vi "读取反控数据解析(子VI).vi"(6 "数据":string, 7 "命令编码CN":string) -> (0 "实时数据发送时间间隔/min":i32=1, 2 "设置超时时间/min":i32=1, 3 "反控命令错误？":bool)   [LabVIEW 2016, in "数据传输系统.lvlib"]
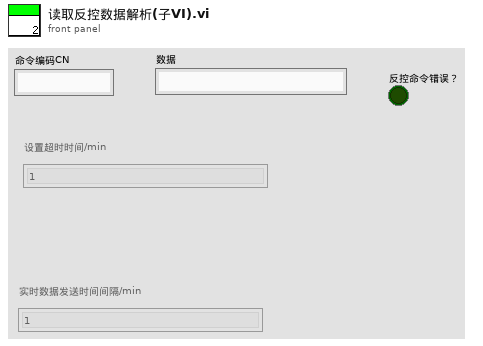
[diagram p1: front panel]
types:
  T1 = enum16{"初始化", "打开连接", "表格比对", "发送数据", "读取数据", "数据处理"}
  T2 = enum16{"CODMn", "CODCr", "氨氮", "总磷", "总氮", "数采仪"}
  T3 = cluster{"高锰酸盐":string, "化学需氧量":string, "氨氮":string, "总磷":string, "总氮":string, "数采仪":string, "高锰酸盐":bool, "化学需氧量":bool, "氨氮":bool, "总磷":bool, "总氮":bool, "数采仪":bool}
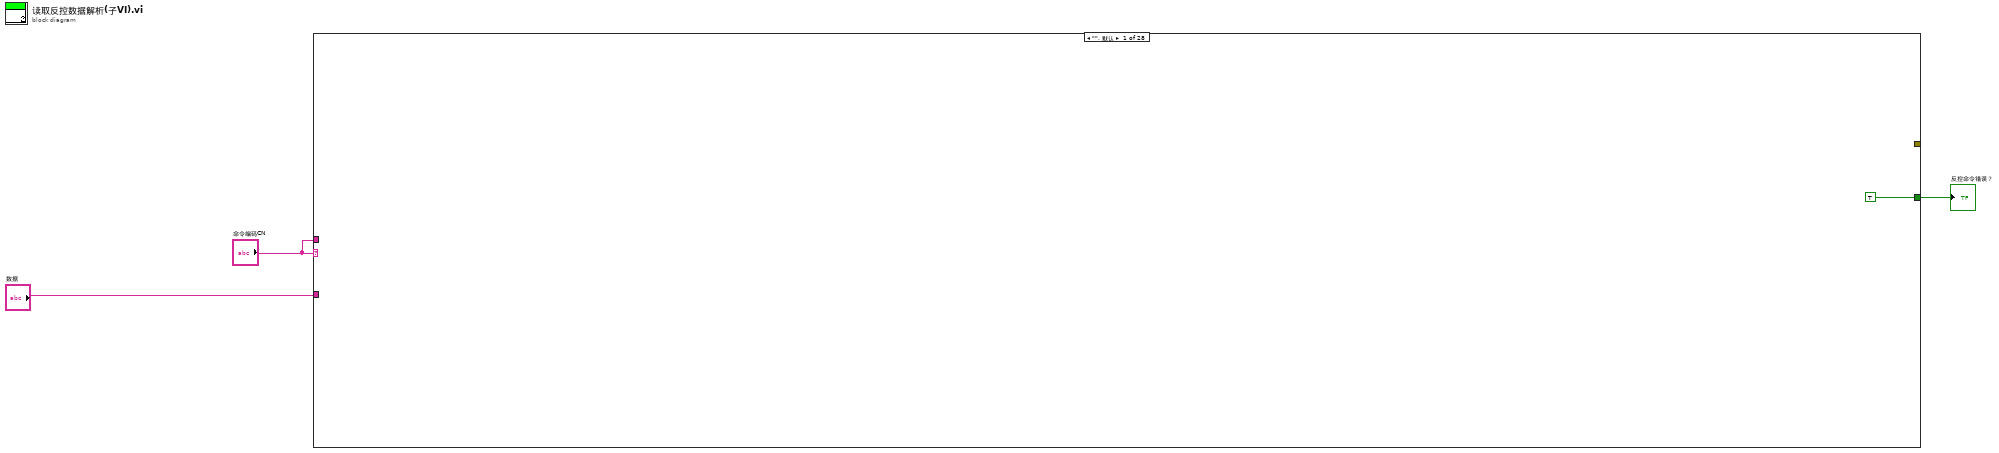
[diagram p0: block diagram]
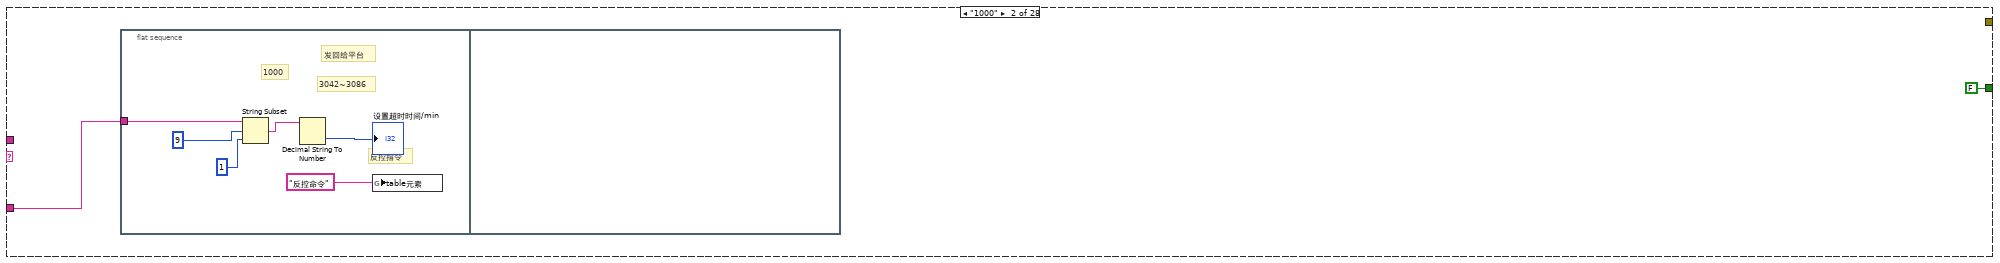
[diagram p2: hidden frame]
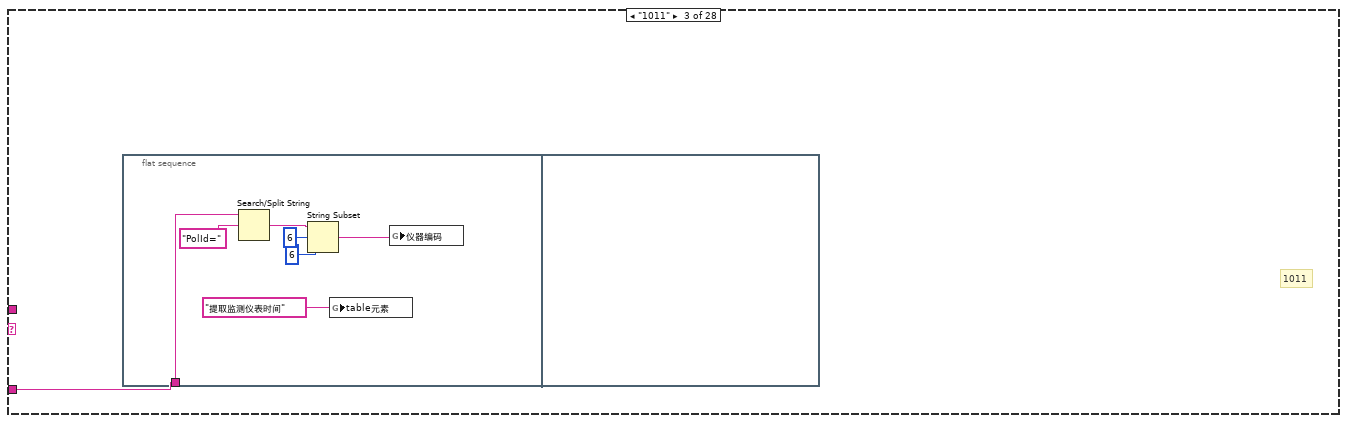
[diagram p3: hidden frame]
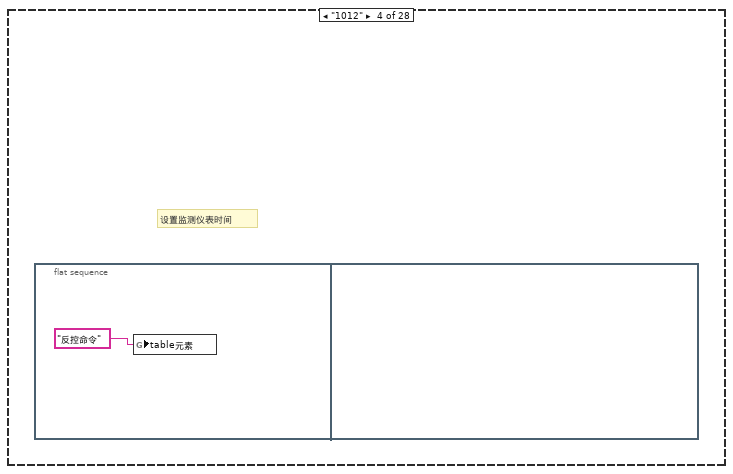
[diagram p4: hidden frame]
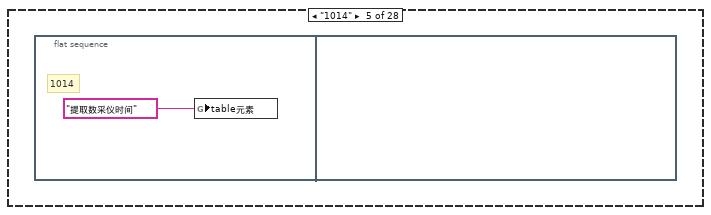
[diagram p5: hidden frame]
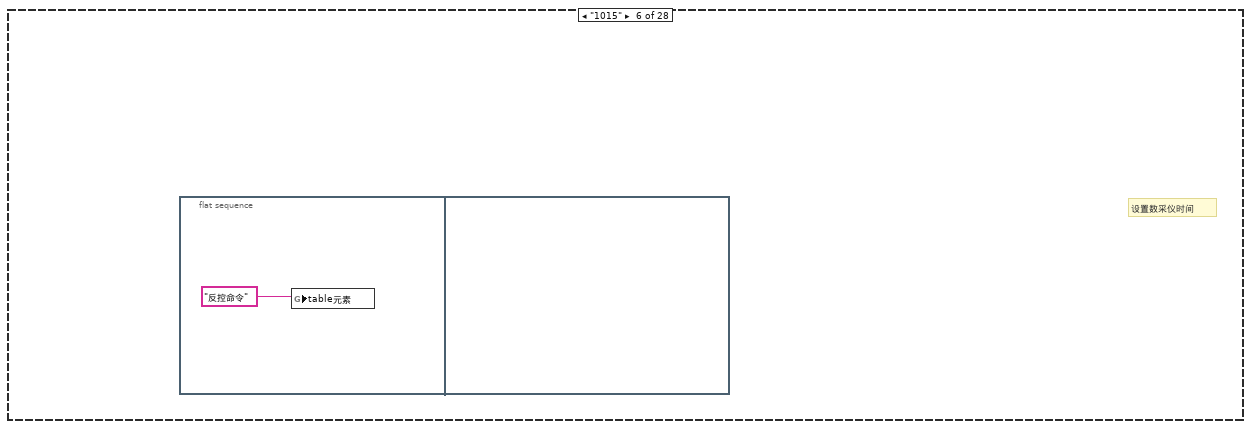
[diagram p6: hidden frame]
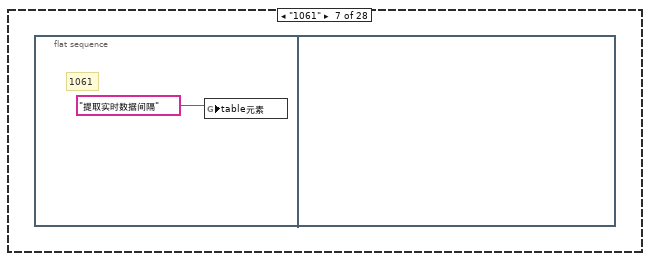
[diagram p7: hidden frame]
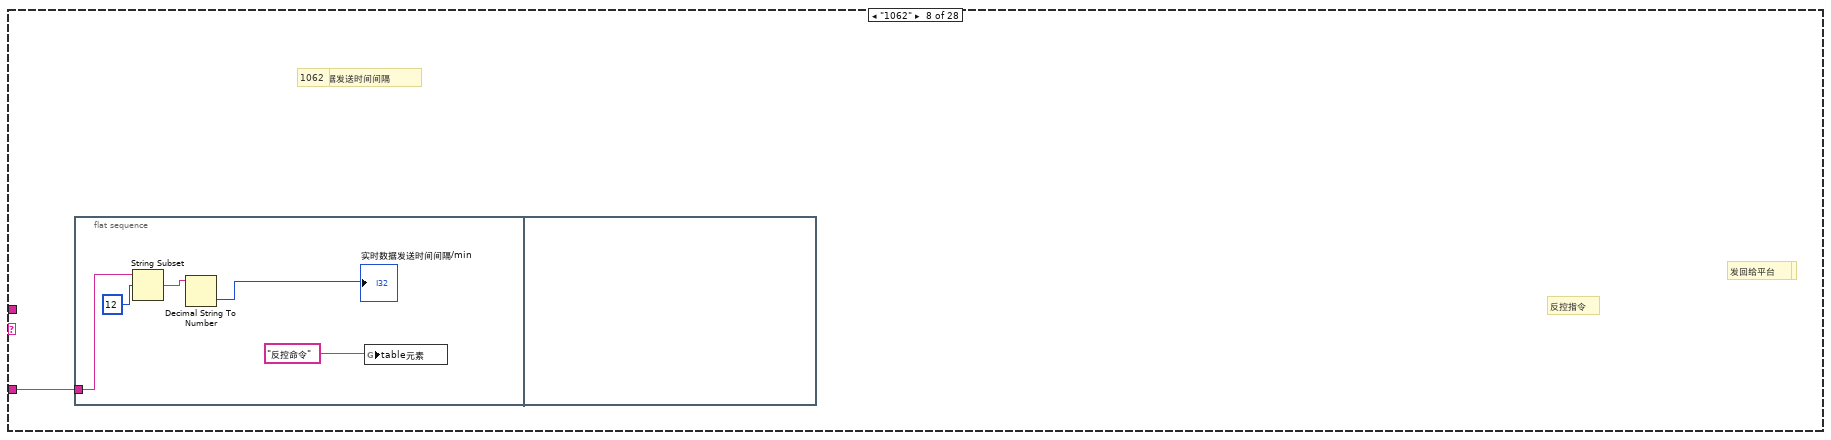
[diagram p8: hidden frame]
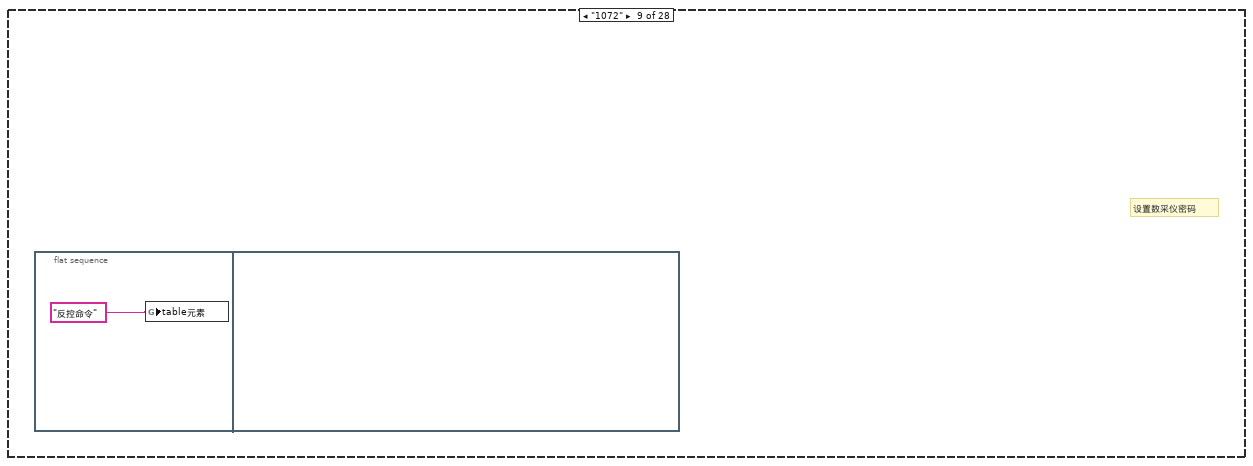
[diagram p9: hidden frame]
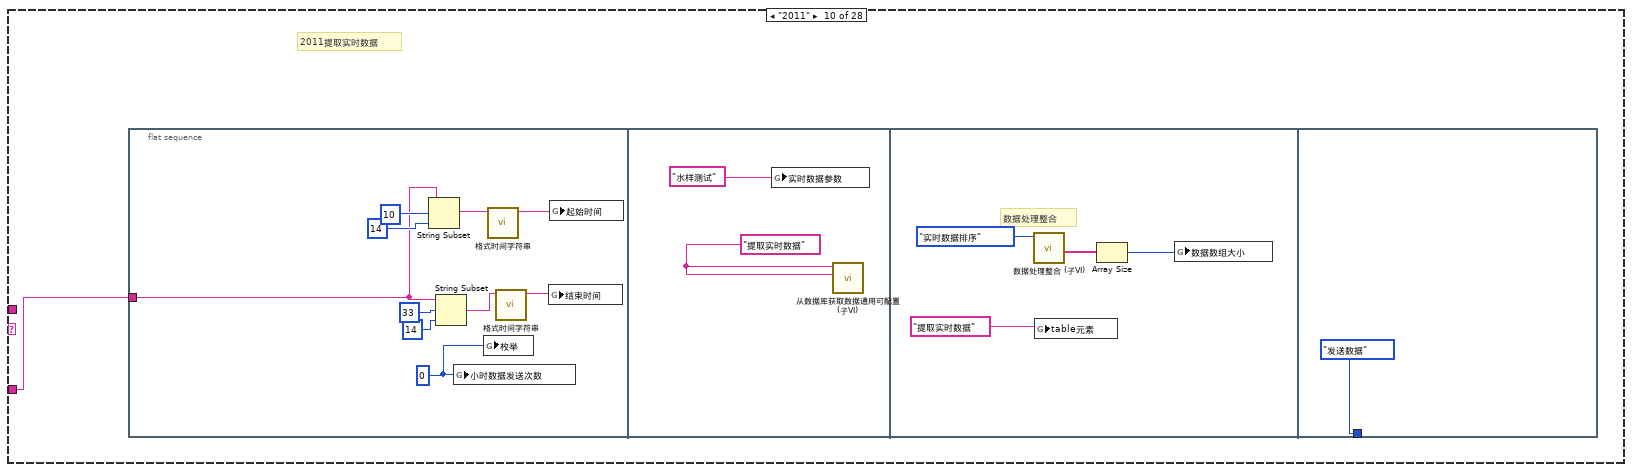
[diagram p10: hidden frame]
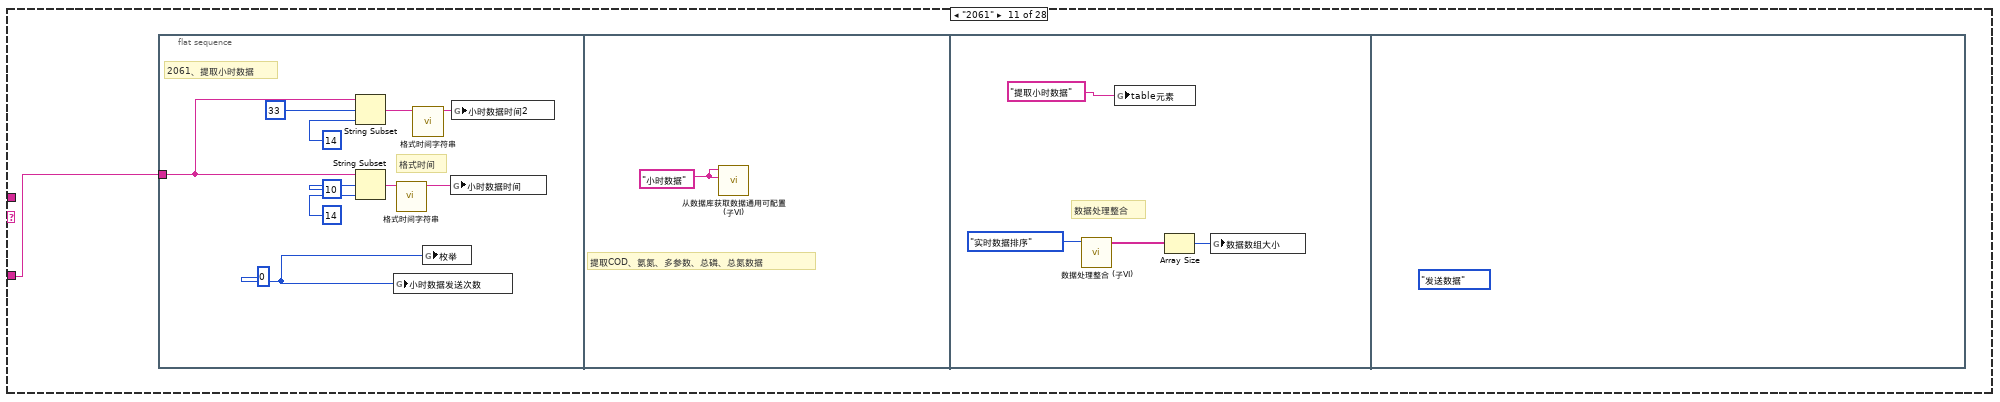
[diagram p11: hidden frame]
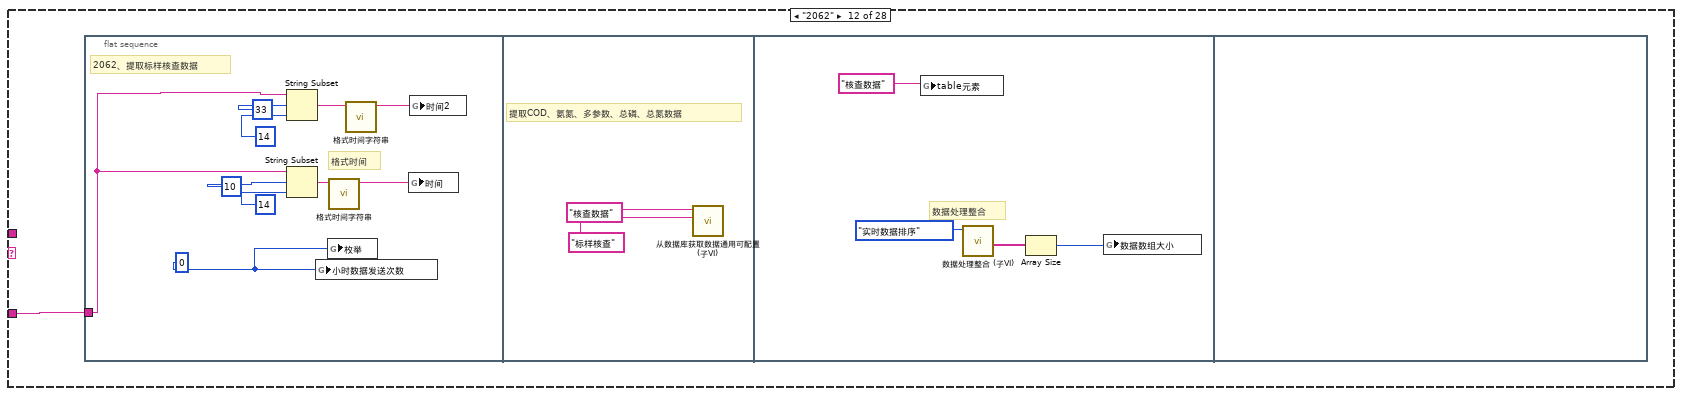
[diagram p12: hidden frame]
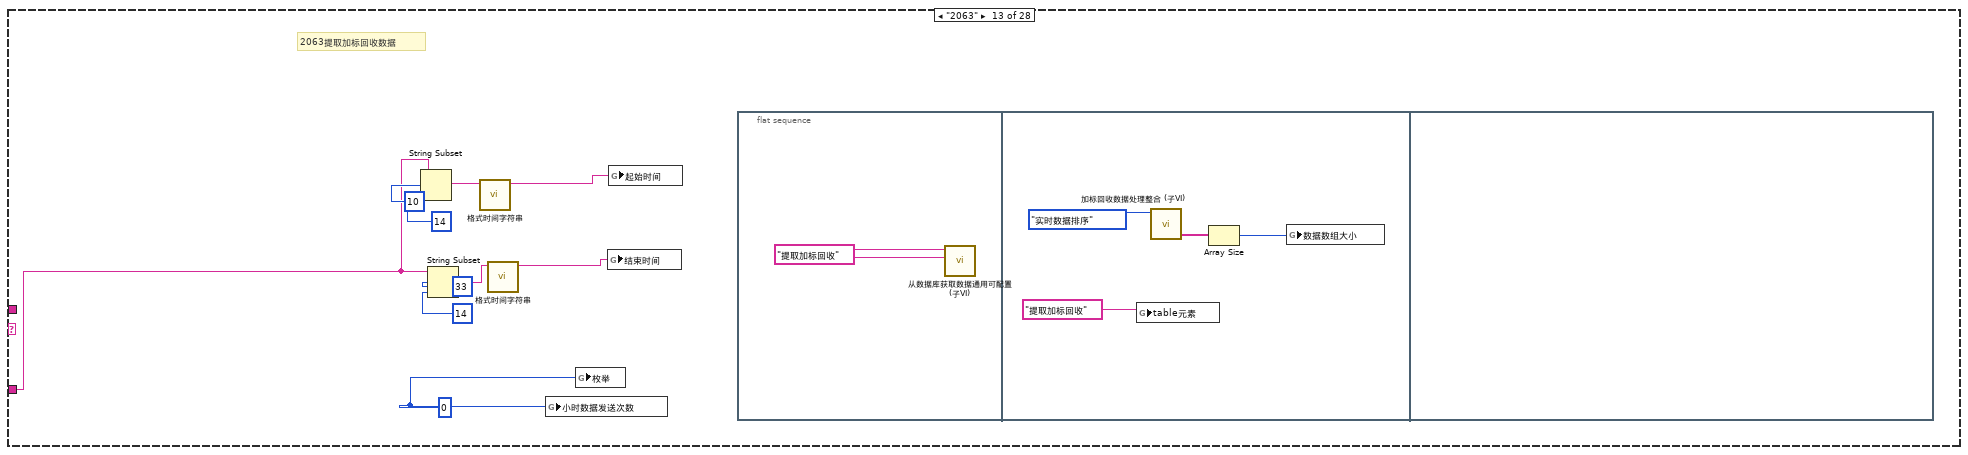
[diagram p13: hidden frame]
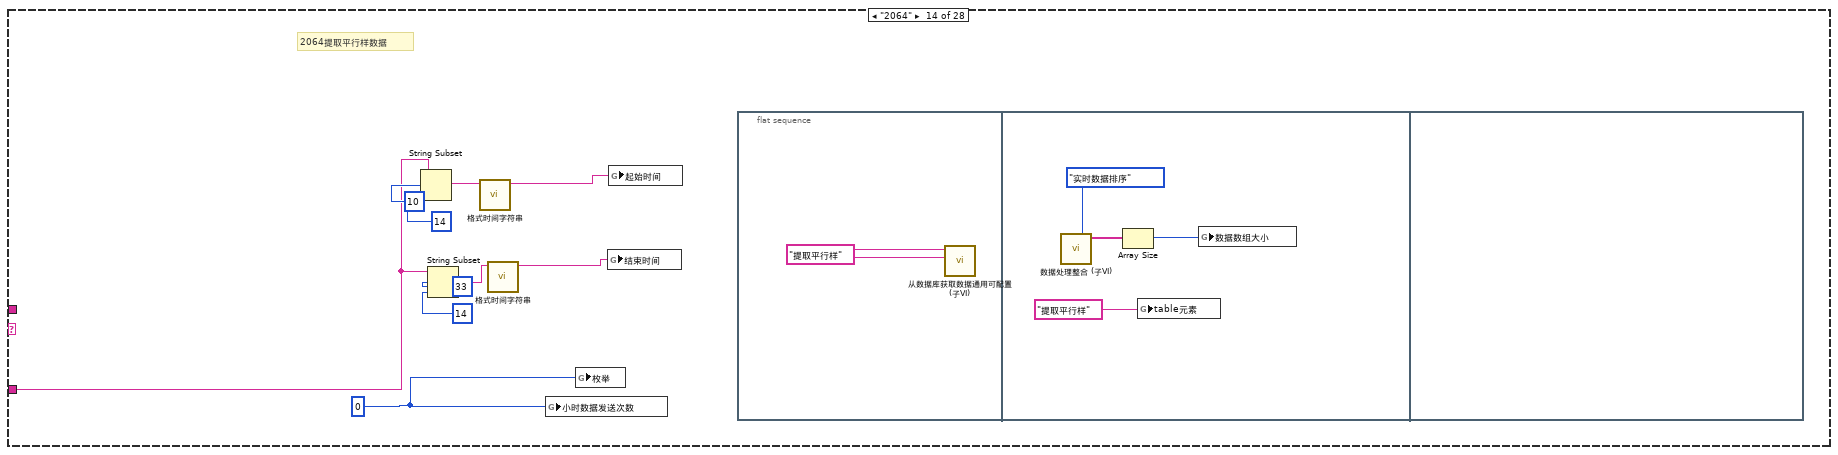
[diagram p14: hidden frame]
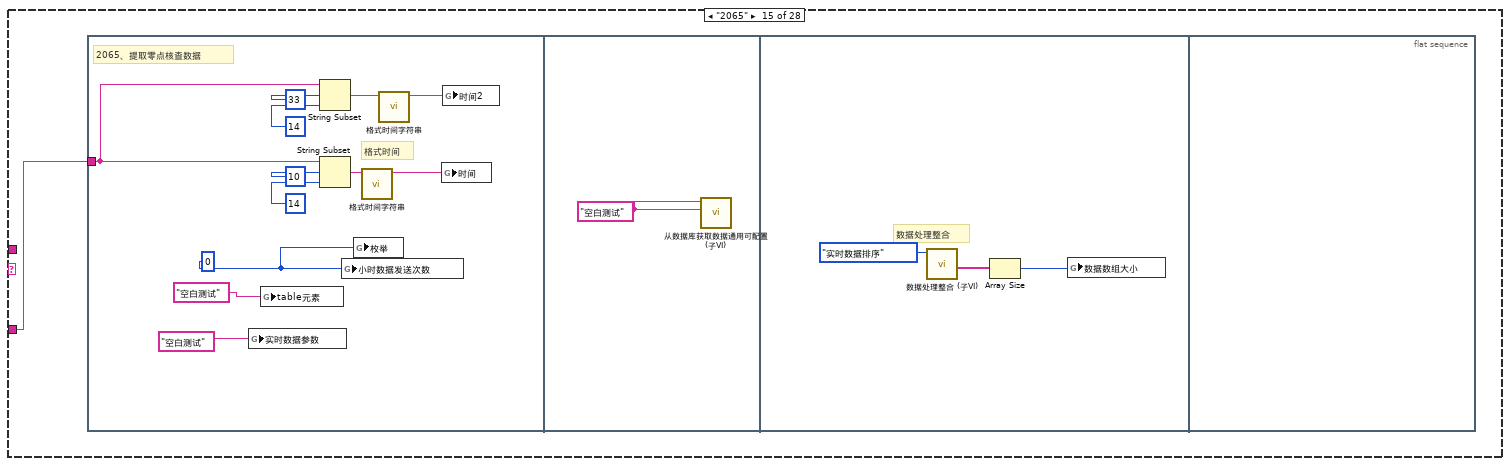
[diagram p15: hidden frame]
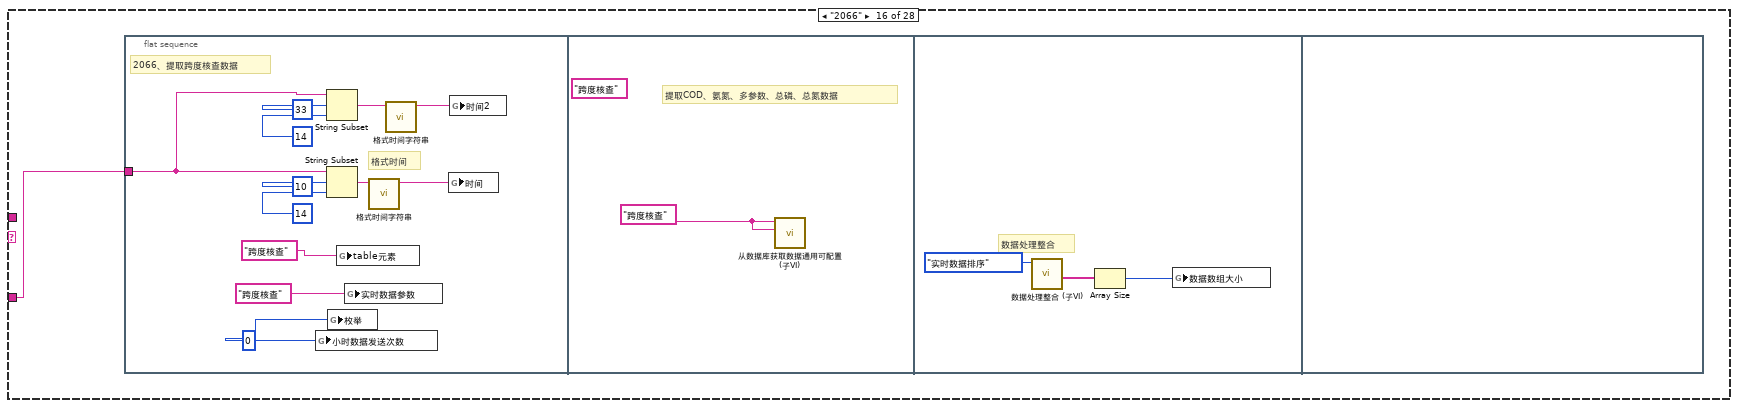
[diagram p16: hidden frame]
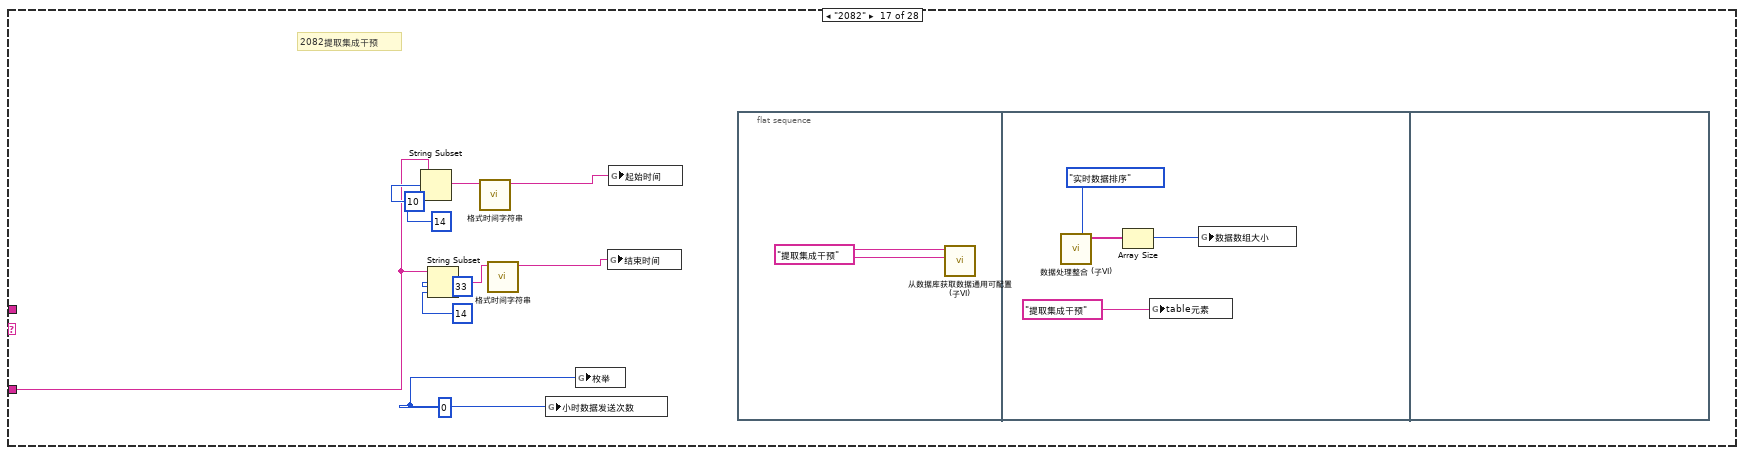
[diagram p17: hidden frame]
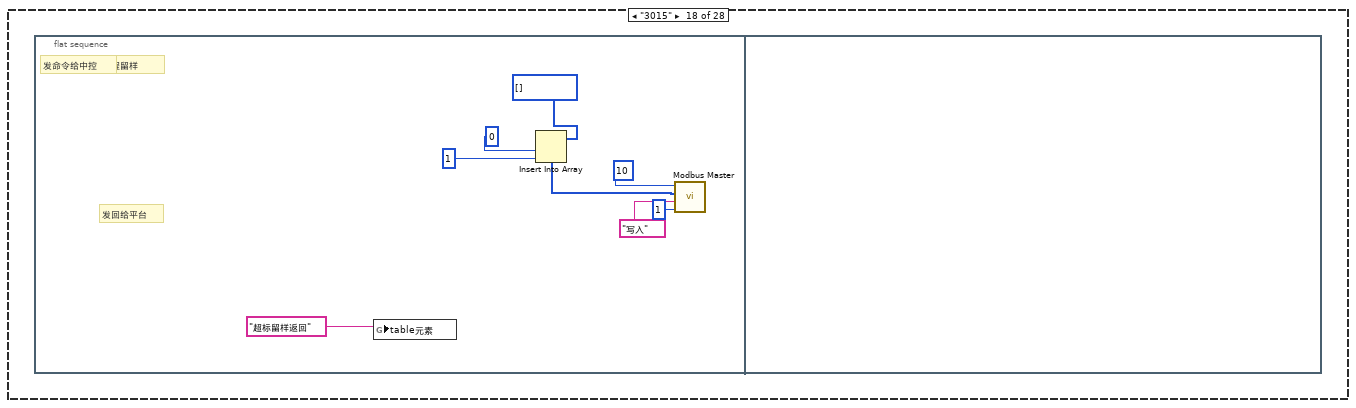
[diagram p18: hidden frame]
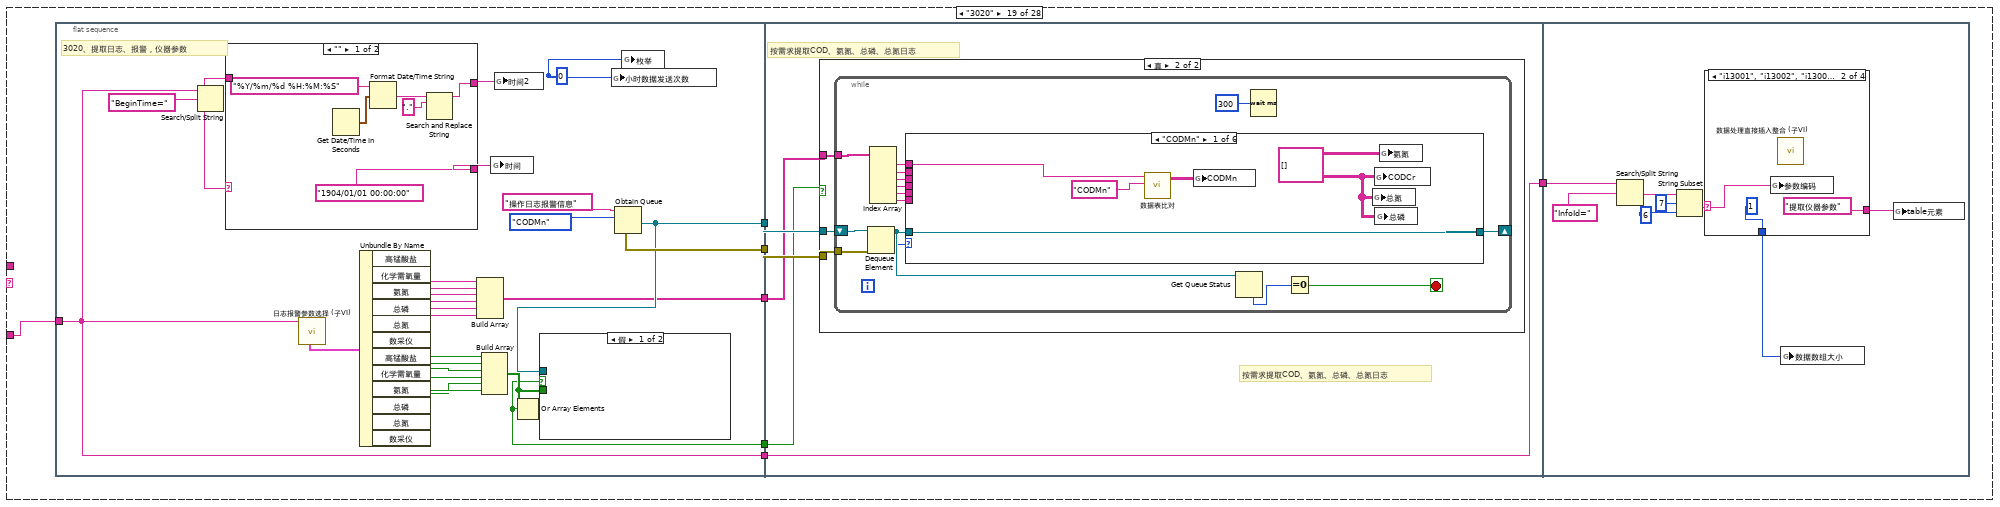
[diagram p19: hidden frame]
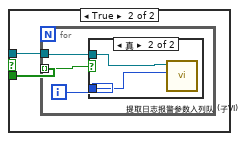
[diagram p20: hidden frame]
diagram:
  n1 = case shown="\"\", 默认" "命令编码CN" {
    tunnel: "命令编码CN" -> [_ _ _ _ _ _ _ _ _ _ _ _ _ _ _ _ _ _ _ _ _ _ _ _ _ _ _ w357]
    tunnel: "数据" -> [_ w6 w13 _ _ _ _ w25 _ w32 w50 w66 w83 w98 w113 w130 w147 _ w172 _ _ _ w299 _ _ _ w339 w354]
    tunnel: [_ _ _ _ _ _ _ _ _ _ _ _ _ _ _ _ _ _ _ _ _ _ _ _ _ _ _ w352] -> _
    tunnel: [TRUE FALSE _ _ _ _ _ _ _ _ _ _ _ _ _ _ _ _ _ _ _ _ _ _ _ _ _ _] -> w1
    frame "", Default {
    }
    frame "1000" {
      n2 = flat-sequence {
        tunnel: w6 -> [w8]
        frame #0 {
          # "发回给平台"
          # "3042~3086"
          # "反控指令"
          # "1000"
          n3 = String Subset(string=w8, offset (0)=9 ("偏移量(0)"), length (rest)=1 ("长度（剩余）")) -> (substring=w10:string)
          n4 = Decimal String To Number(string=w10) -> (number=→"设置超时时间/min":i32)  [unwired: 2 in, 1 out]
          n5 = global write "全局1.vi" "table元素"("反控命令" ("新元素/子数组")) -> ()
        }
        frame #1 {
        }
      }
    }
    frame "1011" {
      # "1011"
      n6 = flat-sequence {
        tunnel: w13 -> [w15]
        frame #0 {
          n7 = Search/Split String(string=w15, search string/char (-)="PolId=" ("搜索字符串/字符(-)")) -> (match + rest of string=w19:string)  [unwired: 1 in, 2 out]
          n8 = String Subset(string=w19, offset (0)=6 ("偏移量(0)"), length (rest)=6 ("长度（剩余）")) -> (substring=w16:string)
          n9 = global write "全局1.vi" "table元素"("提取监测仪表时间") -> ()
          n10 = global write "全局 提取仪器参数.vi" "仪器编码"(w16) -> ()
        }
        frame #1 {
        }
      }
    }
    frame "1012" {
      # "设置监测仪表时间"
      n11 = flat-sequence {
        frame #0 {
          n12 = global write "全局1.vi" "table元素"("反控命令" ("新元素/子数组")) -> ()
        }
        frame #1 {
        }
      }
    }
    frame "1014" {
      n13 = flat-sequence {
        frame #0 {
          # "1014"
          n14 = global write "全局1.vi" "table元素"("提取数采仪时间") -> ()
        }
        frame #1 {
        }
      }
    }
    frame "1015" {
      # "设置数采仪时间"
      n15 = flat-sequence {
        frame #0 {
          n16 = global write "全局1.vi" "table元素"("反控命令" ("新元素/子数组")) -> ()
        }
        frame #1 {
        }
      }
    }
    frame "1061" {
      n17 = flat-sequence {
        frame #0 {
          # "1061"
          n18 = global write "全局1.vi" "table元素"("提取实时数据间隔") -> ()
        }
        frame #1 {
        }
      }
    }
    frame "1062" {
      # "发回给平台"
      # "反控指令"
      # "3042~3086"
      # "设置数据发送时间间隔"
      # "1062"
      n19 = flat-sequence {
        tunnel: w25 -> [w28]
        frame #0 {
          n20 = String Subset(string=w28, offset (0)=12 ("偏移量(0)")) -> (substring=w29:string)  [unwired: 1 in]
          n21 = Decimal String To Number(string=w29) -> (number=→"实时数据发送时间间隔/min":i32)  [unwired: 2 in, 1 out]
          n22 = global write "全局1.vi" "table元素"("反控命令" ("新元素/子数组")) -> ()
        }
        frame #1 {
        }
      }
    }
    frame "1072" {
      # "设置数采仪密码"
      n23 = flat-sequence {
        frame #0 {
          n24 = global write "全局1.vi" "table元素"("反控命令" ("新元素/子数组")) -> ()
        }
        frame #1 {
        }
      }
    }
    frame "2011" {
      # "2011提取实时数据"
      n25 = flat-sequence {
        tunnel: w32 -> [w33]
        tunnel: [T1."发送数据" ("元素")] -> _
        frame #0 {
          w38 = 0 ("数值")
          n26 = String Subset(string=w33, offset (0)=10 ("偏移量(0)"), length (rest)=14 ("长度（剩余）")) -> (substring=w41:string)
          n27 = String Subset(string=w33, offset (0)=33 ("偏移量(0)"), length (rest)=14 ("长度（剩余）")) -> (substring=w39:string)
          n28 = global write "全局 小时数据发送次数.vi" "小时数据发送次数"(w38) -> ()
          n29 = global write "全局1.vi" "枚举"(w38) -> ()
          n30 = call "格式时间字符串.vi"("字符串"=w41) -> ("连接的字符串"=w42:string)  [unwired: 10 in]
          n31 = call "格式时间字符串.vi"("字符串"=w39) -> ("连接的字符串"=w40:string)  [unwired: 10 in]
          n32 = global write "起始时间.vi" "结束时间"(w40) -> ()
          n33 = global write "起始时间.vi" "起始时间"(w42) -> ()
        }
        frame #1 {
          w43 = "提取实时数据" ("新元素/子数组")
          n34 = global write "全局 实时数据参数.vi" "实时数据参数"("水样测试") -> ()
          n35 = call "从数据库获取数据通用可配置(子VI).vi"("table输入"=w43, "列队名（唯一）"=w43) -> ()  [unwired: 8 in, 2 out]
        }
        frame #2 {
          # "数据处理整合"
          n36 = call "数据处理整合 (子VI).vi"("枚举"=enum16{"实时数据排序", "小时数据排序"}."实时数据排序") -> ("已排序的数组"=w47:string[])  [unwired: 10 in]
          n37 = global write "全局1.vi" "table元素"("提取实时数据" ("新元素/子数组")) -> ()
          n38 = Array Size(array=w47) -> (size(s)=w48:i32)
          n39 = global write "全局 数据数组大小.vi" "数据数组大小"(w48) -> ()
        }
        frame #3 {
        }
      }
    }
    frame "2061" {
      n40 = flat-sequence {
        tunnel: w50 -> [w51]
        frame #0 {
          w52 = 0 ("数值")
          # "格式时间"
          # "2061、提取小时数据"
          n41 = String Subset(string=w51, offset (0)=33 ("偏移量(0)"), length (rest)=14 ("长度（剩余）")) -> (substring=w54:string)
          n42 = String Subset(string=w51, offset (0)=10 ("偏移量(0)"), length (rest)=14 ("长度（剩余）")) -> (substring=w55:string)
          n43 = global write "全局 小时数据发送次数.vi" "小时数据发送次数"(w52) -> ()
          n44 = call "格式时间字符串.vi"("字符串"=w55) -> ("连接的字符串"=w56:string)  [unwired: 10 in]
          n45 = call "格式时间字符串.vi"("字符串"=w54) -> ("连接的字符串"=w53:string)  [unwired: 10 in]
          n46 = global write "全局1.vi" "枚举"(w52) -> ()
          n47 = global write "全局 水样时间.vi" "小时数据时间"(w56) -> ()
          n48 = global write "全局 时间2.vi" "小时数据时间2"(w53) -> ()
        }
        frame #1 {
          w61 = "小时数据" ("名称（未命名）")
          # "提取COD、氨氮、多参数、总磷、总氮数据"
          n49 = call "从数据库获取数据通用可配置(子VI).vi"("table输入"=w61, "列队名（唯一）"=w61) -> ()  [unwired: 8 in, 2 out]
        }
        frame #2 {
          # "数据处理整合"
          n50 = call "数据处理整合 (子VI).vi"("枚举"=enum16{"实时数据排序", "小时数据排序"}."实时数据排序") -> ("已排序的数组"=w65:string[])  [unwired: 10 in]
          n51 = global write "全局1.vi" "table元素"("提取小时数据" ("新元素/子数组")) -> ()
          n52 = Array Size(array=w65) -> (size(s)=w64:i32)
          n53 = global write "全局 数据数组大小.vi" "数据数组大小"(w64) -> ()
        }
        frame #3 {
          (unwired) T1."发送数据" ("元素")
        }
      }
    }
    frame "2062" {
      n54 = flat-sequence {
        tunnel: w66 -> [w67]
        frame #0 {
          w68 = 0 ("数值")
          # "格式时间"
          # "2062、提取标样核查数据"
          n55 = String Subset(string=w67, offset (0)=33 ("偏移量(0)"), length (rest)=14 ("长度（剩余）")) -> (substring=w70:string)
          n56 = String Subset(string=w67, offset (0)=10 ("偏移量(0)"), length (rest)=14 ("长度（剩余）")) -> (substring=w71:string)
          n57 = global write "全局 小时数据发送次数.vi" "小时数据发送次数"(w68) -> ()
          n58 = global write "全局1.vi" "枚举"(w68) -> ()
          n59 = call "格式时间字符串.vi"("字符串"=w71) -> ("连接的字符串"=w72:string)  [unwired: 10 in]
          n60 = call "格式时间字符串.vi"("字符串"=w70) -> ("连接的字符串"=w69:string)  [unwired: 10 in]
          n61 = global write "全局 水样时间.vi" "时间"(w72) -> ()
          n62 = global write "全局 时间2.vi" "时间2"(w69) -> ()
        }
        frame #1 {
          # "提取COD、氨氮、多参数、总磷、总氮数据"
          n63 = call "从数据库获取数据通用可配置(子VI).vi"("table输入"="标样核查" ("新元素/子数组"), "列队名（唯一）"="核查数据" ("新元素/子数组")) -> ()  [unwired: 8 in, 2 out]
        }
        frame #2 {
          # "数据处理整合"
          n64 = global write "全局1.vi" "table元素"("核查数据" ("新元素/子数组")) -> ()
          n65 = call "数据处理整合 (子VI).vi"("枚举"=enum16{"实时数据排序", "小时数据排序"}."实时数据排序") -> ("已排序的数组"=w81:string[])  [unwired: 10 in]
          n66 = Array Size(array=w81) -> (size(s)=w82:i32)
          n67 = global write "全局 数据数组大小.vi" "数据数组大小"(w82) -> ()
        }
        frame #3 {
        }
      }
    }
    frame "2063" {
      w88 = 0 ("数值")
      # "2063提取加标回收数据"
      n68 = String Subset(string=w83, offset (0)=10 ("偏移量(0)"), length (rest)=14 ("长度（剩余）")) -> (substring=w85:string)
      n69 = String Subset(string=w83, offset (0)=33 ("偏移量(0)"), length (rest)=14 ("长度（剩余）")) -> (substring=w87:string)
      n70 = call "格式时间字符串.vi"("字符串"=w85) -> ("连接的字符串"=w84:string)  [unwired: 10 in]
      n71 = call "格式时间字符串.vi"("字符串"=w87) -> ("连接的字符串"=w86:string)  [unwired: 10 in]
      n72 = global write "全局 小时数据发送次数.vi" "小时数据发送次数"(w88) -> ()
      n73 = global write "全局1.vi" "枚举"(w88) -> ()
      n74 = global write "起始时间.vi" "结束时间"(w86) -> ()
      n75 = global write "起始时间.vi" "起始时间"(w84) -> ()
      n76 = flat-sequence {
        frame #0 {
          w93 = "提取加标回收" ("新元素/子数组")
          n77 = call "从数据库获取数据通用可配置(子VI).vi"("table输入"=w93, "列队名（唯一）"=w93) -> ()  [unwired: 8 in, 2 out]
        }
        frame #1 {
          n78 = global write "全局1.vi" "table元素"("提取加标回收" ("新元素/子数组")) -> ()
          n79 = call "加标回收数据处理整合 (子VI).vi"("枚举"=enum16{"实时数据排序", "小时数据排序"}."实时数据排序") -> ("已排序的数组"=w95:string[])  [unwired: 10 in]
          n80 = Array Size(array=w95) -> (size(s)=w97:i32)
          n81 = global write "全局 数据数组大小.vi" "数据数组大小"(w97) -> ()
        }
        frame #2 {
        }
      }
    }
    frame "2064" {
      w103 = 0 ("数值")
      # "2064提取平行样数据"
      n82 = String Subset(string=w98, offset (0)=10 ("偏移量(0)"), length (rest)=14 ("长度（剩余）")) -> (substring=w100:string)
      n83 = String Subset(string=w98, offset (0)=33 ("偏移量(0)"), length (rest)=14 ("长度（剩余）")) -> (substring=w102:string)
      n84 = call "格式时间字符串.vi"("字符串"=w100) -> ("连接的字符串"=w99:string)  [unwired: 10 in]
      n85 = call "格式时间字符串.vi"("字符串"=w102) -> ("连接的字符串"=w101:string)  [unwired: 10 in]
      n86 = global write "全局 小时数据发送次数.vi" "小时数据发送次数"(w103) -> ()
      n87 = global write "全局1.vi" "枚举"(w103) -> ()
      n88 = global write "起始时间.vi" "结束时间"(w101) -> ()
      n89 = global write "起始时间.vi" "起始时间"(w99) -> ()
      n90 = flat-sequence {
        frame #0 {
          w108 = "提取平行样" ("新元素/子数组")
          n91 = call "从数据库获取数据通用可配置(子VI).vi"("table输入"=w108, "列队名（唯一）"=w108) -> ()  [unwired: 8 in, 2 out]
        }
        frame #1 {
          n92 = call "数据处理整合 (子VI).vi"("枚举"=enum16{"实时数据排序", "小时数据排序"}."实时数据排序") -> ("已排序的数组"=w112:string[])  [unwired: 10 in]
          n93 = Array Size(array=w112) -> (size(s)=w111:i32)
          n94 = global write "全局1.vi" "table元素"("提取平行样" ("新元素/子数组")) -> ()
          n95 = global write "全局 数据数组大小.vi" "数据数组大小"(w111) -> ()
        }
        frame #2 {
        }
      }
    }
    frame "2065" {
      n96 = flat-sequence {
        tunnel: w113 -> [w115]
        frame #0 {
          w116 = 0 ("数值")
          # "格式时间"
          # "2065、提取零点核查数据"
          n97 = global write "全局 实时数据参数.vi" "实时数据参数"("空白测试" ("新元素/子数组")) -> ()
          n98 = global write "全局1.vi" "table元素"("空白测试" ("新元素/子数组")) -> ()
          n99 = String Subset(string=w115, offset (0)=33 ("偏移量(0)"), length (rest)=14 ("长度（剩余）")) -> (substring=w119:string)
          n100 = String Subset(string=w115, offset (0)=10 ("偏移量(0)"), length (rest)=14 ("长度（剩余）")) -> (substring=w120:string)
          n101 = global write "全局 小时数据发送次数.vi" "小时数据发送次数"(w116) -> ()
          n102 = global write "全局1.vi" "枚举"(w116) -> ()
          n103 = call "格式时间字符串.vi"("字符串"=w120) -> ("连接的字符串"=w121:string)  [unwired: 10 in]
          n104 = call "格式时间字符串.vi"("字符串"=w119) -> ("连接的字符串"=w118:string)  [unwired: 10 in]
          n105 = global write "全局 水样时间.vi" "时间"(w121) -> ()
          n106 = global write "全局 时间2.vi" "时间2"(w118) -> ()
        }
        frame #1 {
          w126 = "空白测试" ("新元素/子数组")
          n107 = call "从数据库获取数据通用可配置(子VI).vi"("table输入"=w126, "列队名（唯一）"=w126) -> ()  [unwired: 8 in, 2 out]
        }
        frame #2 {
          # "数据处理整合"
          n108 = call "数据处理整合 (子VI).vi"("枚举"=enum16{"实时数据排序", "小时数据排序"}."实时数据排序") -> ("已排序的数组"=w128:string[])  [unwired: 10 in]
          n109 = Array Size(array=w128) -> (size(s)=w129:i32)
          n110 = global write "全局 数据数组大小.vi" "数据数组大小"(w129) -> ()
        }
        frame #3 {
        }
      }
    }
    frame "2066" {
      n111 = flat-sequence {
        tunnel: w130 -> [w132]
        frame #0 {
          w133 = 0 ("数值")
          # "格式时间"
          # "2066、提取跨度核查数据"
          n112 = global write "全局 小时数据发送次数.vi" "小时数据发送次数"(w133) -> ()
          n113 = String Subset(string=w132, offset (0)=33 ("偏移量(0)"), length (rest)=14 ("长度（剩余）")) -> (substring=w136:string)
          n114 = String Subset(string=w132, offset (0)=10 ("偏移量(0)"), length (rest)=14 ("长度（剩余）")) -> (substring=w137:string)
          n115 = global write "全局1.vi" "枚举"(w133) -> ()
          n116 = global write "全局1.vi" "table元素"("跨度核查" ("新元素/子数组")) -> ()
          n117 = global write "全局 实时数据参数.vi" "实时数据参数"("跨度核查" ("新元素/子数组")) -> ()
          n118 = call "格式时间字符串.vi"("字符串"=w137) -> ("连接的字符串"=w138:string)  [unwired: 10 in]
          n119 = call "格式时间字符串.vi"("字符串"=w136) -> ("连接的字符串"=w135:string)  [unwired: 10 in]
          n120 = global write "全局 水样时间.vi" "时间"(w138) -> ()
          n121 = global write "全局 时间2.vi" "时间2"(w135) -> ()
        }
        frame #1 {
          w143 = "跨度核查" ("新元素/子数组")
          (unwired) "跨度核查" ("名称（未命名）")
          # "提取COD、氨氮、多参数、总磷、总氮数据"
          n122 = call "从数据库获取数据通用可配置(子VI).vi"("table输入"=w143, "列队名（唯一）"=w143) -> ()  [unwired: 8 in, 2 out]
        }
        frame #2 {
          # "数据处理整合"
          n123 = call "数据处理整合 (子VI).vi"("枚举"=enum16{"实时数据排序", "小时数据排序"}."实时数据排序") -> ("已排序的数组"=w146:string[])  [unwired: 10 in]
          n124 = Array Size(array=w146) -> (size(s)=w145:i32)
          n125 = global write "全局 数据数组大小.vi" "数据数组大小"(w145) -> ()
        }
        frame #3 {
        }
      }
    }
    frame "2082" {
      w152 = 0 ("数值")
      # "2082提取集成干预"
      n126 = String Subset(string=w147, offset (0)=10 ("偏移量(0)"), length (rest)=14 ("长度（剩余）")) -> (substring=w149:string)
      n127 = String Subset(string=w147, offset (0)=33 ("偏移量(0)"), length (rest)=14 ("长度（剩余）")) -> (substring=w151:string)
      n128 = call "格式时间字符串.vi"("字符串"=w149) -> ("连接的字符串"=w148:string)  [unwired: 10 in]
      n129 = call "格式时间字符串.vi"("字符串"=w151) -> ("连接的字符串"=w150:string)  [unwired: 10 in]
      n130 = global write "全局 小时数据发送次数.vi" "小时数据发送次数"(w152) -> ()
      n131 = global write "全局1.vi" "枚举"(w152) -> ()
      n132 = global write "起始时间.vi" "结束时间"(w150) -> ()
      n133 = global write "起始时间.vi" "起始时间"(w148) -> ()
      n134 = flat-sequence {
        frame #0 {
          w157 = "提取集成干预" ("新元素/子数组")
          n135 = call "从数据库获取数据通用可配置(子VI).vi"("table输入"=w157, "列队名（唯一）"=w157) -> ()  [unwired: 8 in, 2 out]
        }
        frame #1 {
          n136 = call "数据处理整合 (子VI).vi"("枚举"=enum16{"实时数据排序", "小时数据排序"}."实时数据排序") -> ("已排序的数组"=w161:string[])  [unwired: 10 in]
          n137 = Array Size(array=w161) -> (size(s)=w160:i32)
          n138 = global write "全局1.vi" "table元素"("提取集成干预" ("新元素/子数组")) -> ()
          n139 = global write "全局 数据数组大小.vi" "数据数组大小"(w160) -> ()
        }
        frame #2 {
        }
      }
    }
    frame "3015" {
      n140 = flat-sequence {
        frame #0 {
          # "发命令给中控"
          # "发回给平台"
          # "3015、手动远程留样"
          n141 = global write "全局1.vi" "table元素"("超标留样返回" ("新元素/子数组")) -> ()
          n142 = Insert Into Array(array=u16[] [] ("holding register values"), index=0 ("索引"), new element=u16 1 ("新元素/子数组")) -> (w165:u16[])
          n143 = call "Modbus Master.vi"("Unit ID"=u8 1, "读取写入选择"="写入", "holding register values"=w165, "starting address"=u16 10) -> ()  [unwired: 6 in, 2 out]
        }
        frame #1 {
        }
      }
    }
    frame "3020" {
      n144 = flat-sequence {
        tunnel: [w181] -> w176
        tunnel: [w182] -> w175
        tunnel: [w180] -> w174
        tunnel: [w178] -> w173
        tunnel: w172 -> [w177]
        tunnel: [w177] -> w170
        tunnel: w176 -> [w229]
        tunnel: w175 -> [w228]
        tunnel: w174 -> [w227]
        tunnel: w173 -> [w226]
        tunnel: [w225] -> w171
        tunnel: w170 -> [w225]
        tunnel: w171 -> [w277]
        frame #0 {
          w200 = 0 ("数值")
          # "3020、提取日志、报警，仪器参数"
          n145 = Search/Split String(string=w177, search string/char (-)="BeginTime=" ("搜索字符串")) -> (match + rest of string=w199:string)  [unwired: 1 in, 2 out]
          n146 = case shown="\"\"" w199 {
            tunnel: ["1904/01/01 00:00:00" w222] -> w202
            tunnel: w199 -> [_ w216]
            tunnel: [w210 w217] -> w198
            frame "" {
              n147 = Get Date/Time In Seconds() -> (seconds since 1Jan1904=w212:timestamp)
              n148 = Format Date/Time String(time format string (%c)="%Y/%m/%d %H:%M:%S" ("时间格式字符串(%c)"), seconds (now)=w212) -> (date/time string=w213:string)  [unwired: 1 in]
              n149 = Search and Replace String(input string=w213, search string="." ("搜索字符串")) -> (result string=w210:string)  [unwired: 6 in, 3 out]
            }
            frame "真", Default {
              # "格式时间"
              n150 = String Subset(string=w216, offset (0)=33 ("偏移量(0)"), length (rest)=14 ("长度（剩余）")) -> (substring=w220:string)
              n151 = String Subset(string=w216, offset (0)=10 ("偏移量(0)"), length (rest)=14 ("长度（剩余）")) -> (substring=w221:string)
              n152 = call "格式时间字符串.vi"("字符串"=w220) -> ("连接的字符串"=w217:string)  [unwired: 10 in]
              n153 = call "格式时间字符串.vi"("字符串"=w221) -> ("连接的字符串"=w222:string)  [unwired: 10 in]
            }
          }
          n154 = call "日志报警参数选择 (子VI).vi"("String输入"=w177) -> ("输出簇"=w185:T3)  [unwired: 9 in, 1 out]
          n155 = Unbundle By Name(w185) -> ("高锰酸盐"=w192:string, "化学需氧量"=w193:string, "氨氮"=w194:string, "总磷"=w195:string, "总氮"=w196:string, "数采仪"=w197:string, "高锰酸盐"=w186:bool, "化学需氧量"=w187:bool, "氨氮"=w188:bool, "总磷"=w189:bool, "总氮"=w190:bool, "数采仪"=w191:bool)
          n156 = Build Array(w192, w193, w194, w195, w196, w197) -> (w180:string[])
          n157 = Build Array(w186, w187, w188, w189, w190, w191) -> (w179:bool[])
          n158 = global write "全局 水样时间.vi" "时间"(w202) -> ()
          n159 = global write "全局 时间2.vi" "时间2"(w198) -> ()
          n160 = Or Array Elements(Boolean array=w179) -> (logical OR=w178:bool)
          n161 = global write "全局 小时数据发送次数.vi" "小时数据发送次数"(w200) -> ()
          n162 = Obtain Queue(name (unnamed)="操作日志报警信息" ("名称（未命名）"), element data type=T2."CODMn") -> (queue out=w181:refnum<queue>, error out=w182:errorcluster)  [unwired: 3 in, 1 out]
          n163 = case shown="假" w178 {
            tunnel: w181 -> [_ w204]
            tunnel: w179 -> [_ w203]
            frame False {
            }
            frame True {
              n164 = for {
                tunnel: w203 -> [w206] mode=indexing
                tunnel: w204 -> [w205]
                i -> [w207]
                n165 = case shown="真" w206 {
                  tunnel: w207 -> [_ w209]
                  tunnel: w205 -> [_ w208]
                  frame False {
                  }
                  frame True {
                    n166 = call "提取日志报警参数入列队 (子VI).vi"("枚举"=w209, "queue in"=w208) -> ()  [unwired: 10 in]
                  }
                }
              }
            }
          }
          n167 = global write "全局1.vi" "枚举"(w200) -> ()
        }
        frame #1 {
          # "按需求提取COD、氨氮、总磷、总氮日志"
          # "按需求提取COD、氨氮、总磷、总氮日志"
          n168 = case shown="真" w226 {
            tunnel: w228 -> [_ w232]
            tunnel: w229 -> [_ w231]
            tunnel: w227 -> [_ w230]
            frame False {
            }
            frame True {
              n169 = while {
                shift-right: [w246] -> _
                shift-left: w231 -> [w247]
                tunnel: w232 -> [w245]
                tunnel: w230 -> [w240]
                stop <- w242 stop-if-true
                n170 = Dequeue Element(queue=w247, error in (no error)=w245) -> (queue out=w244:refnum<queue>, element=w239:T2)  [unwired: 1 in, 2 out]
                n171 = Index Array(array=w240) -> (element #1=w238:string, element #2=w237:string, element #3=w236:string, element #4=w235:string, element #5=w234:string, element #6=w233:string)  [unwired: 6 in]
                n172 = case shown="\"CODMn\"" w239 {
                  tunnel: w244 -> [w252 _ w261 w266 w270 w275]
                  tunnel: [w252 _ w261 w266 w270 w275] -> w246
                  tunnel: w238 -> [w249 _ _ _ _ _]
                  tunnel: w237 -> [_ w254 _ _ _ _]
                  tunnel: w236 -> [_ _ w258 _ _ _]
                  tunnel: w235 -> [_ _ _ w263 _ _]
                  tunnel: w234 -> [_ _ _ _ w268 _]
                  tunnel: w233 -> [_ _ _ _ _ w272]
                  frame "CODMn" {
                    w248 = string[][] [] ("氨氮")
                    n173 = call "数据表比对.vi"("仪器日志参数"="CODMn" ("元素"), "table输入"=w249) -> ("待发送数据"=w250:string[][])  [unwired: 7 in, 2 out]
                    n174 = global write "全局 所有参数.vi" "CODMn"(w250) -> ()
                    n175 = global write "全局 所有参数.vi" "总氮"(w248) -> ()
                    n176 = global write "全局 所有参数.vi" "CODCr"(w248) -> ()
                    n177 = global write "全局 所有参数.vi" "总磷"(w248) -> ()
                    n178 = global write "全局 所有参数.vi" "氨氮"(w248) -> ()
                  }
                  frame "CODCr" {
                    w253 = string[][] [] ("氨氮")
                    n179 = call "数据表比对.vi"("仪器日志参数"="CODCr" ("元素"), "table输入"=w254) -> ("待发送数据"=w255:string[][])  [unwired: 7 in, 2 out]
                    n180 = global write "全局 所有参数.vi" "CODCr"(w255) -> ()
                    n181 = global write "全局 所有参数.vi" "CODMn"(w253) -> ()
                    n182 = global write "全局 所有参数.vi" "总氮"(w253) -> ()
                    n183 = global write "全局 所有参数.vi" "总磷"(w253) -> ()
                    n184 = global write "全局 所有参数.vi" "氨氮"(w253) -> ()
                  }
                  frame "氨氮" {
                    w257 = string[][] [] ("氨氮")
                    n185 = call "数据表比对.vi"("仪器日志参数"="氨氮" ("元素"), "table输入"=w258) -> ("待发送数据"=w259:string[][])  [unwired: 7 in, 2 out]
                    n186 = global write "全局 所有参数.vi" "氨氮"(w259) -> ()
                    n187 = global write "全局 所有参数.vi" "CODMn"(w257) -> ()
                    n188 = global write "全局 所有参数.vi" "总氮"(w257) -> ()
                    n189 = global write "全局 所有参数.vi" "CODCr"(w257) -> ()
                    n190 = global write "全局 所有参数.vi" "总磷"(w257) -> ()
                  }
                  frame "总磷" {
                    w262 = string[][] [] ("氨氮")
                    n191 = call "数据表比对.vi"("仪器日志参数"="总磷" ("元素"), "table输入"=w263) -> ("待发送数据"=w264:string[][])  [unwired: 7 in, 2 out]
                    n192 = global write "全局 所有参数.vi" "总磷"(w264) -> ()
                    n193 = global write "全局 所有参数.vi" "CODMn"(w262) -> ()
                    n194 = global write "全局 所有参数.vi" "总氮"(w262) -> ()
                    n195 = global write "全局 所有参数.vi" "CODCr"(w262) -> ()
                    n196 = global write "全局 所有参数.vi" "氨氮"(w262) -> ()
                  }
                  frame "总氮" {
                    w267 = string[][] [] ("氨氮")
                    n197 = call "数据表比对.vi"("仪器日志参数"="总氮" ("元素"), "table输入"=w268) -> ("待发送数据"=w269:string[][])  [unwired: 7 in, 2 out]
                    n198 = global write "全局 所有参数.vi" "总氮"(w269) -> ()
                    n199 = global write "全局 所有参数.vi" "CODMn"(w267) -> ()
                    n200 = global write "全局 所有参数.vi" "氨氮"(w267) -> ()
                    n201 = global write "全局 所有参数.vi" "CODCr"(w267) -> ()
                    n202 = global write "全局 所有参数.vi" "总磷"(w267) -> ()
                  }
                  frame "数采仪" {
                    n203 = call "数据表比对.vi"("仪器日志参数"="系统" ("元素"), "table输入"=w272) -> ("待发送数据"=w273:string[][])  [unwired: 7 in, 2 out]
                    n204 = global write "全局 所有参数.vi" "DO"(w273) -> ()
                  }
                }
                n205 = Get Queue Status(queue=w244) -> (# elements in queue=w243:i32)  [unwired: 2 in, 7 out]
                n206 = Wait (ms)(milliseconds to wait=u32 300 ("等待时间（毫秒）")) -> ()  [unwired: 1 out]
                n207 = Equal To 0?(x=w243) -> (x = 0?=w242:bool)
              }
            }
          }
        }
        frame #2 {
          n208 = Search/Split String(string=w277, search string/char (-)="InfoId=" ("搜索字符串/字符(-)")) -> (match + rest of string=w282:string)  [unwired: 1 in, 2 out]
          n209 = String Subset(string=w282, offset (0)=7 ("偏移量(0)"), length (rest)=6 ("长度（剩余）")) -> (substring=w279:string)
          n210 = case shown="\"i13001\", \"i13002\", \"i13003\", \"i13004\", \"i13005\", \"i13006\", \"i13007\", \"i13008\", \"i13009\", \"i13010\", \"i13011\", \"i13012\", \"i13013\"" w279 {
            selector: w279 -> [_ w288 _ _]
            tunnel: ["操作日志" ("名称（未命名）") "提取仪器参数" ("名称（未命名）") "报警信息" ("名称（未命名）") "" ("名称（未命名）")] -> w276
            tunnel: [w284 1 ("数据数组大小") w291 _] -> w278
            frame "i11001", "i21001" {
              # "数据处理整合"
              # "i11001日志"
              n211 = call "数据处理整合 (子VI).vi"("枚举"=enum16{"实时数据排序", "小时数据排序"}."实时数据排序") -> ("已排序的数组"=w285:string[])  [unwired: 10 in]
              n212 = Array Size(array=w285) -> (size(s)=w284:i32)
            }
            frame "i13001", "i13002", "i13003", "i13004", "i13005", "i13006", "i13007", "i13008", "i13009", "i13010", "i13011", "i13012", "i13013" {
              n213 = global write "全局 提取仪器参数.vi" "参数编码"(w288) -> ()
              n214 = call "数据处理直接插入整合 (子VI).vi"() -> ()  [unwired: 12 in]
            }
            frame "i12001" {
              # "数据处理整合"
              # "i12001状态"
              n215 = call "数据处理整合 (子VI).vi"("枚举"=enum16{"实时数据排序", "小时数据排序"}."实时数据排序") -> ("已排序的数组"=w292:string[])  [unwired: 10 in]
              n216 = Array Size(array=w292) -> (size(s)=w291:i32)
            }
            frame Default {
            }
          }
          n217 = global write "全局 数据数组大小.vi" "数据数组大小"(w278) -> ()
          n218 = global write "全局1.vi" "table元素"(w276) -> ()
        }
      }
    }
    frame "3021" {
      n219 = flat-sequence {
        frame #0 {
          # "设置仪表参数"
          n220 = global write "全局1.vi" "table元素"("反控命令" ("新元素/子数组")) -> ()
        }
        frame #1 {
        }
      }
    }
    frame "3040" {
      # "提取现场系统信息（3040）"
      n221 = flat-sequence {
        frame #0 {
          n222 = global write "全局1.vi" "table元素"("提取现场系统信息" ("新元素/子数组")) -> ()
        }
        frame #1 {
        }
      }
    }
    frame "3041" {
      # "提取现场经纬度及环境信息（3041）"
      n223 = flat-sequence {
        frame #0 {
          n224 = call "获取环境参数 (子VI).vi"() -> ()  [unwired: 12 in]
          n225 = global write "全局1.vi" "table元素"("提取经纬度环境信息" ("新元素/子数组")) -> ()
        }
        frame #1 {
        }
      }
    }
    frame "3042" {
      n226 = flat-sequence {
        tunnel: w299 -> [w301]
        frame #0 {
          # "反控指令"
          # "反控指令\n切换运行模式"
          # "发命令给中控"
          # "0维护，1常规，2应急，3质控"
          n227 = Search/Split String(string=w301, search string/char (-)="RunMode" ("搜索字符串/字符(-)")) -> (match + rest of string=w312:string)  [unwired: 1 in, 2 out]
          n228 = String Subset(string=w312, offset (0)=8 ("偏移量(0)"), length (rest)=1 ("长度（剩余）")) -> (substring=w309:string)
          n229 = case shown="\"2\"" w309 {
            tunnel: [u16 0 ("新元素/子数组") u16 1 ("新元素/子数组") u16 2 ("新元素/子数组") u16 3 ("新元素/子数组")] -> w305
            frame "0", Default {
            }
            frame "1" {
            }
            frame "2" {
            }
            frame "3" {
            }
          }
          n230 = global write "全局1.vi" "table元素"("反控命令" ("新元素/子数组")) -> ()
          n231 = Insert Into Array(array=u16[] [] ("holding register values"), index=0 ("索引"), new element=w305) -> (w306:u16[])
          n232 = call "Modbus Master.vi"("Unit ID"=u8 1, "读取写入选择"="写入", "holding register values"=w306, "starting address"=u16 0) -> ()  [unwired: 6 in, 2 out]
        }
        frame #1 {
        }
      }
    }
    frame "3043" {
      # "远程重启数采仪"
      n233 = flat-sequence {
        frame #0 {
          n234 = global write "全局1.vi" "table元素"("反控命令" ("新元素/子数组")) -> ()
        }
        frame #1 {
        }
      }
    }
    frame "3044" {
      n235 = flat-sequence {
        frame #0 {
          # "反控指令"
          # "发命令给中控"
          n236 = call "Modbus Master.vi"("Unit ID"=u8 1, "读取写入选择"="写入", "holding register values"=u16[] [1], "starting address"=u16 2) -> ()  [unwired: 6 in, 2 out]
        }
        frame #1 {
          # "反控指令\n单次测量"
          n237 = Wait (ms)(milliseconds to wait=u32 500 ("等待时间（毫秒）")) -> ()  [unwired: 1 out]
        }
        frame #2 {
          n238 = global write "全局1.vi" "table元素"("反控命令" ("新元素/子数组")) -> ()
          n239 = call "Modbus Master.vi"("Unit ID"=u8 1, "读取写入选择"="写入", "holding register values"=u16[] [0], "starting address"=u16 2) -> ()  [unwired: 6 in, 2 out]
        }
        frame #3 {
        }
      }
    }
    frame "3045", "3046" {
      n240 = flat-sequence {
        frame #0 {
          # "发命令给中控"
          n241 = call "Modbus Master.vi"("Unit ID"=u8 1, "读取写入选择"="写入", "holding register values"=u16[] [1], "starting address"=u16 3) -> ()  [unwired: 6 in, 2 out]
        }
        frame #1 {
          # "反控指令"
          # "反控指令\n急停"
          # "3045"
          n242 = Wait (ms)(milliseconds to wait=u32 500 ("等待时间（毫秒）")) -> ()  [unwired: 1 out]
        }
        frame #2 {
          n243 = global write "全局1.vi" "table元素"("反控命令" ("新元素/子数组")) -> ()
          n244 = call "Modbus Master.vi"("Unit ID"=u8 1, "读取写入选择"="写入", "holding register values"=u16[] [0], "starting address"=u16 3) -> ()  [unwired: 6 in, 2 out]
        }
        frame #3 {
        }
      }
    }
    frame "3056" {
      n245 = flat-sequence {
        tunnel: w339 -> [w341]
        frame #0 {
          # "发回给平台"
          # "设置测量时间间隔"
          # "发命令给中控"
          n246 = Search/Split String(string=w341, search string/char (-)="RunInterval" ("搜索字符串/字符(-)")) -> (match + rest of string=w348:string)  [unwired: 1 in, 2 out]
          n247 = Decimal String To Number(string=w348, offset=12 ("偏移量(0)")) -> (number=w344:i32)  [unwired: 1 in, 1 out]
          n248 = Insert Into Array(array=u16[] [] ("holding register values"), index=0 ("索引"), new element=w344) -> (w343:u16[])
          n249 = global write "全局1.vi" "table元素"("反控命令" ("新元素/子数组")) -> ()
          n250 = call "Modbus Master.vi"("Unit ID"=u8 1, "读取写入选择"="写入", "holding register values"=w343, "starting address"=u16 14) -> ()  [unwired: 6 in, 2 out]
        }
        frame #1 {
        }
      }
    }
    frame "3080", "3081", "3082", "3083", "3084", "3085", "3086" {
      n251 = flat-sequence {
        tunnel: w357 -> [w361]
        tunnel: [w359] -> w356
        tunnel: w354 -> [w358]
        tunnel: w356 -> [w386]
        tunnel: [w386] -> w355
        tunnel: w355 -> [w391]
        tunnel: [w388] -> w353
        tunnel: [w394] -> w352
        tunnel: w353 -> [w394]
        frame #0 {
          # "30 启动标液核查  1CODmn  2 氨氮  3总磷  4总氮  5CODCr\n31 加标回收\n32 平行样测试\n33 零点核查\n34 跨度核查\n35 校零\n36 校标"
          # "1CODmn  2 氨氮  3总磷  4总氮  5CODCr"
          # "启动单台仪器标液核查"
          # "发命令给中控"
          n252 = Search/Split String(string=w358, search string/char (-)="PolId" ("搜索字符串/字符(-)")) -> (match + rest of string=w366:string)  [unwired: 1 in, 2 out]
          n253 = String Subset(string=w366, offset (0)=6 ("偏移量(0)"), length (rest)=6 ("长度（剩余）")) -> (substring=w363:string)
          n254 = case shown="\"w01019\"" w363 {
            tunnel: [0 ("长度（剩余）") 1 ("长度（剩余）") 2 ("长度（剩余）") 3 ("长度（剩余）") 4 ("长度（剩余）") 5 ("长度（剩余）")] -> w362
            frame "", Default {
            }
            frame "w01019" {
            }
            frame "w21003" {
            }
            frame "w21011" {
            }
            frame "w21001" {
            }
            frame "w01018" {
            }
          }
          n255 = Insert Into Array(array=u16[] [] ("holding register values"), index=0 ("索引"), new element=w362) -> (w367:u16[])
          n256 = case shown="\"3086\"" w361 {
            tunnel: [u16 99 ("starting address") u16 30 ("starting address") u16 31 ("starting address") u16 32 ("starting address") u16 33 ("starting address") u16 34 ("starting address") u16 35 ("starting address") u16 36 ("starting address")] -> w359
            frame "", Default {
            }
            frame "3080" {
            }
            frame "3081" {
            }
            frame "3082" {
            }
            frame "3083" {
            }
            frame "3084" {
            }
            frame "3085" {
            }
            frame "3086" {
            }
          }
          n257 = call "Modbus Master.vi"("Unit ID"=u8 1, "读取写入选择"="写入", "holding register values"=w367, "starting address"=w359) -> ()  [unwired: 6 in, 2 out]
        }
        frame #1 {
          n258 = Wait (ms)(milliseconds to wait=u32 500 ("等待时间（毫秒）")) -> ()  [unwired: 1 out]
        }
        frame #2 {
          n259 = global write "全局1.vi" "table元素"("反控命令" ("新元素/子数组")) -> ()
          n260 = call "Modbus Master.vi"("Unit ID"=u8 1, "读取写入选择"="写入", "holding register values"=u16[] [0], "starting address"=w391) -> ("error out"=w388:errorcluster)  [unwired: 6 in, 1 out]
        }
        frame #3 {
        }
      }
    }
  }
  "反控命令错误？" <- w1
